vi "Initialise.vi"(8 "error in (no error)":errorcluster, 10 "Message in":refnum<class "InitialiseMessage.lvclass">, 11 "MeritFactor in":refnum<class "MeritFactor.lvclass">) -> (0 "error out":errorcluster, 3 "MeritFactor out":refnum<class "MeritFactor.lvclass">)   [LabVIEW 2012, in "MeritFactor.lvclass"]
doc: "This method is called when an initialise message is received. It mainly initialises the RabbitMQ connectivity. \n\nOverride this method when your component needs special initialisation (e.g. of software or hardware resources). In that case, don't forget to call the parent for proper implementation. If your component owns subcomponents, they count as resources, so you have to initialise them by calling their own initialise functions"
uses:
  MeritFactor.lvclass
  <vilib>/Distrio/Murmex/InitialiseMessage/InitialiseMessage.lvclass
  <vilib>/Distrio/Murmex/Murmex/Murmex.lvclass
  MeritFactor.lvclass/MeritFactor.ctl
panel:
  # "This method is called when the INTIALISE\ntrigger is sent. \n\nOverride this method when your component needs to\nrespond to this trigger. \n\nCall parent for proper implementation"
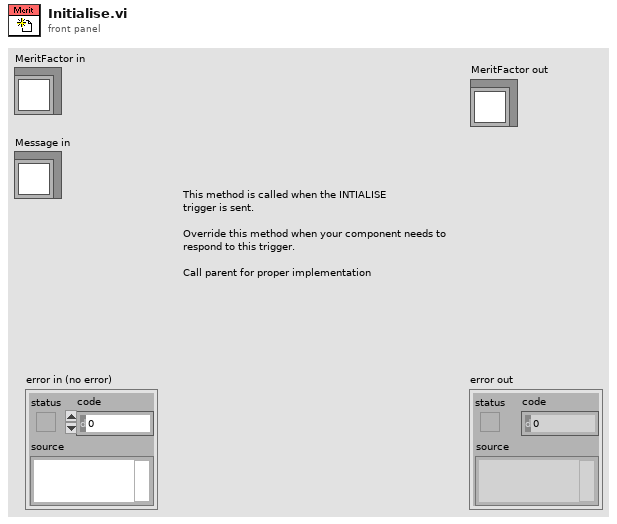
[diagram p1: front panel]
types:
  T1 = typedef "Image Type" = u32
  T2 = typedef "IMAQ Image.ctl" = refnum<image>
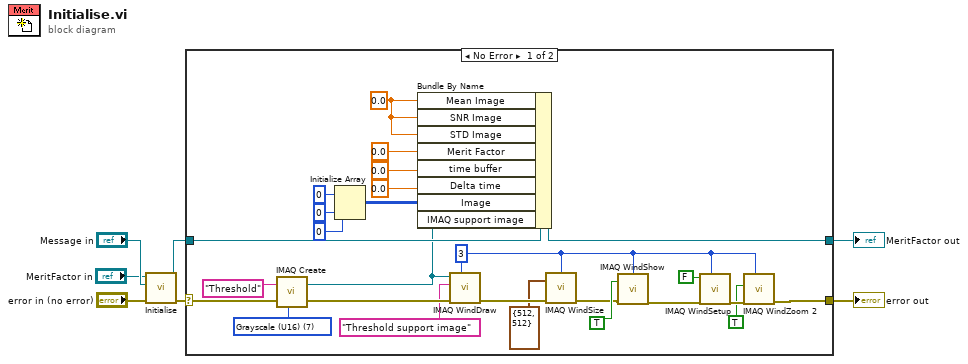
[diagram p0: block diagram]
diagram:
  n1 = call-parent "Initialise.vi"("error in (no error)"="error in (no error)", "Message in"="Message in", "Murmex in"="MeritFactor in") -> ("error out"=w4:errorcluster, "Murmex out"=w3:refnum<class "MeritFactor.lvclass">)  [unwired: 7 in]
  n2 = case shown="No Error" w4 {
    selector: w4 -> [w23 w34]
    tunnel: w3 -> [w26 w35]
    tunnel: [w25 w35] -> w2
    tunnel: [w11 w34] -> w1
    frame No Error {
      w9 = 3 ("Window Number (0...15)")
      w21 = T1 7 items=["Grayscale (U8)", "Grayscale (I16)", "Grayscale (SGL)", "Complex (CSG)", "RGB (U32)", "HSL (U32)", "RGB (U64)", "Grayscale (U16)"] ("Image Type")
      w24 = sgl 0.0 ("run-time cluster.Mean Image")
      n3 = call "IMAQ Create"("Image Name"="Threshold", "Image Type"=w21, "error in (no error)"=w23) -> ("New Image"=w19:T2, "error out"=w20:errorcluster)  [unwired: 2 in]
      n4 = Initialize Array(u16 0 ("element"), 0 ("dimension size"), 0 ("dimension size")) -> (w33:u16[][])
      n5 = Bundle By Name(cluster=w26, "Mean Image"=w24, "SNR Image"=w24, "STD Image"=w24, "Merit Factor"=0.0 ("settings cluster.Merit Factor"), "time buffer"=0.0 ("run-time cluster.time buffer"), "Delta time"=0.0 ("run-time cluster.Delta time"), "Image"=w33, "IMAQ support image"=w19) -> (w25:refnum<class "MeritFactor.lvclass">)
      n6 = call "IMAQ WindDraw"("Window Number (0...15)"=w9, "error in (no error)"=w20, "Title"="Threshold support image", "Image"=w19) -> ("error out"=w17:errorcluster)  [unwired: 6 in, 1 out]
      n7 = call "IMAQ WindSize"("error in (no error)"=w17, "Width & Height"=cluster{"Width":i32, "Height":i32} {"Width"=512, "Height"=512}, "Window Number"=w9) -> ("error out"=w10:errorcluster)  [unwired: 3 in, 2 out]
      n8 = call "IMAQ WindShow"("error in (no error)"=w10, "Hide/Show (Show)"=TRUE, "Window Number (0...15)"=w9) -> ("error out"=w14:errorcluster)  [unwired: 3 in, 2 out]
      n9 = call "IMAQ WindSetup"("Window Number (0...15)"=w9, "error in (no error)"=w14, "Window can grow? (Yes)"=FALSE) -> ("error out"=w13:errorcluster)  [unwired: 8 in]
      n10 = call "IMAQ WindZoom 2"("Window Number (0...15)"=w9, "error in (no error)"=w13, "Zoom to Fit? (False)"=TRUE) -> ("error out"=w11:errorcluster)  [unwired: 5 in, 3 out]
    }
    frame Error {
    }
  }
  "error out" <- w1
  "MeritFactor out" <- w2
